vi "Get Event Reference.vi"(4 "error in (no error)":errorcluster) -> (0 "error out":errorcluster, 3 "System Error":refnum<user-event>)   [LabVIEW 2015, in "ude_Handle Errors.lvlib"]
uses:
  ude_Handle Errors.lvlib
  Event Data.ctl
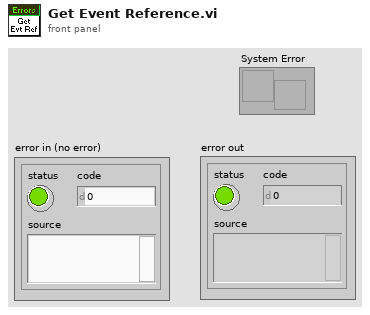
[diagram p1: front panel]
types:
  T1 = typedef "ude_Handle Errors.lvlib/Event Data.ctl" = cluster{"Error Data":errorcluster}
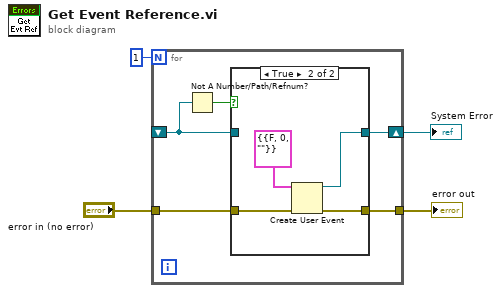
[diagram p0: block diagram]
diagram:
  n1 = for {
    N: 1 -> [_]
    shift-right: [w6] -> w4
    shift-left: _ -> [w8]
    tunnel: "error in (no error)" -> [w7]
    tunnel: [w5] -> w1
    n2 = Not A Number/Path/Refnum?(number/path/refnum=w8) -> (NaN/Path/Refnum?=w9:bool)
    n3 = case shown="True" w9 {
      tunnel: w8 -> [w11 _]
      tunnel: w7 -> [w10 w15]
      tunnel: [w11 w14] -> w6
      tunnel: [w10 w13] -> w5
      frame False {
      }
      frame True {
        n4 = Create User Event(user event datatype=T1 {"Error Data"={"status"=FALSE, "code"=0, "source"=""}} ("data"), error in=w15) -> (user event=w14:refnum<user-event>, error out=w13:errorcluster)
      }
    }
  }
  "error out" <- w1
  "System Error" <- w4
